vi "trio_open.vi"(8 "error in":errorcluster, 11 "Host IP":string="192.168.1.250") -> (0 "error out":errorcluster, 3 "reference out":refnum<k7>)   [LabVIEW 2024]
uses:
  <instrlib>/Trio Motion/Trio Motion Library.lvlib
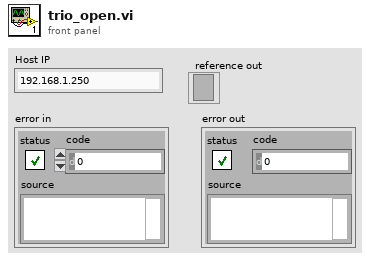
[diagram p1: front panel]
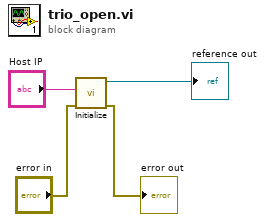
[diagram p0: block diagram]
diagram:
  n1 = call <instrlib>:"Initialize.vi"("error in (no error)"="error in", "strHost"="Host IP") -> ("error out"=→"error out":errorcluster, "reference out"=→"reference out":refnum<k7>)  [unwired: 7 in, 1 out]
